vi "Wait for Next Streaming Buffer.vi"(8 "error in (no error)":errorcluster, 9 "Timeout (ms) Default: 10000":i32=10000, 10 "Buffer in":refnum<class "Buffer.lvclass">, 11 "Camera in":refnum<class "Camera.lvclass">) -> (0 "error out":errorcluster, 2 "Buffer":refnum<class "Buffer.lvclass">, 3 "Camera":refnum<class "Camera.lvclass">)   [LabVIEW 2020, in "Camera.lvclass"]
doc: "Waits for a new frame to be captured and return the captured frame as a buffer.\n\nReturns an <b>Error 56</b> if no new frame is received within the specificed timeout."
uses:
  Camera.lvclass
  Buffer/Buffer.lvclass
  Camera.lvclass/Camera.ctl
  Buffer/Buffer.lvclass/Buffer.ctl
  bin/gindustrialcam_32-1.dll
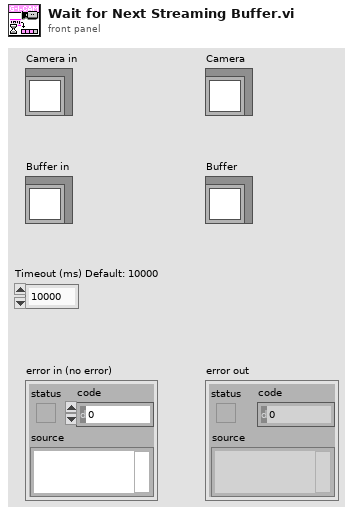
[diagram p1: front panel]
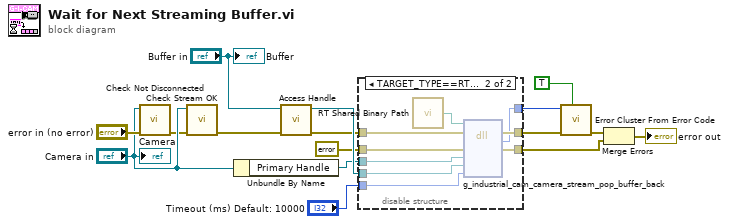
[diagram p0: block diagram]
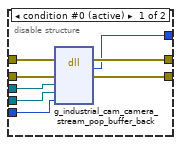
[diagram p2: hidden frame]
diagram:
  n1 = call "Check Not Disconnected.vi"("error in (no error)"="error in (no error)", "Camera in"="Camera in") -> ("error out"=w1:errorcluster)  [unwired: 9 in]
  n2 = call "Check Stream OK.vi"("error in (no error)"=w1, "Camera in"="Camera in") -> ("error out"=w11:errorcluster)  [unwired: 9 in]
  n3 = Unbundle By Name("Camera in") -> ("Primary Handle"=w9:refnum<data-value>)
  n4 = call "Access Handle.vi"("error in (no error)"=w11, "Buffer"="Buffer in") -> ("error out"=w15:errorcluster, "Handle"=w16:refnum<data-value>)  [unwired: 8 in]
  n5 = disable-structure shown="TARGET_TYPE==RT&&OS==Linux" {
    disable-tunnel: w16 -> [w24 w33]
    disable-tunnel: w15 -> [w23 w32]
    disable-tunnel: "Timeout (ms) Default: 10000" -> [w22 w31]
    disable-tunnel: w9 -> [w21 w30]
    disable-tunnel: [w20 w29] -> w8
    disable-tunnel: [w19 w28] -> w7
    disable-tunnel: errorcluster {"status"=FALSE, "code"=0, "source"=""} ("error constant") -> [w18 w27]
    disable-tunnel: [w17 w26] -> w3
    frame condition #0 (active) {
      n6 = dll-call lib="C:/serenial/lib/g-industrial-camera/LabVIEW/g_industrial_cam/bin/gindustrialcam_*-1.*" fn="g_industrial_cam_camera_stream_pop_buffer_back"(error in=w23, "err"=w18, "cam_edvr"=w21, "buffer_edvr"=w24, "timeout_ms"=w22) -> (error out=w20:errorcluster, "Mg_Error"=w19:i32, "err"=w17:errorcluster)  [unwired: 5 in, 1 out]
    }
    frame condition #1 {
      n7 = call "RT Shared Binary Path.vi"() -> ("Path"=w25:path)
      n8 = dll-call lib="?" fn="g_industrial_cam_camera_stream_pop_buffer_back" ("gindustrialcam_*-1.*:g_industrial_cam_camera_stream_pop_buffer")(path in=w25, error in=w32, "err"=w27, "cam_edvr"=w30, "buffer_edvr"=w33, "timeout_ms"=w31) -> (error out=w29:errorcluster, "Mg_Error"=w28:i32, "err"=w26:errorcluster)  [unwired: 4 in, 1 out]
    }
  }
  n9 = call <vilib>:"Error Cluster From Error Code.vi"("show call chain? (False)"=TRUE, "error in (no error)"=w8, "error code (0)"=w7) -> ("error out"=w6:errorcluster)  [unwired: 6 in]
  n10 = Merge Errors(w6, w3) -> (→"error out":errorcluster)
  "Camera" <- "Camera in"
  "Buffer" <- "Buffer in"
